vi "MCP4725_with_GraphforLoop.vi"() -> ()   [LabVIEW 2017]
uses:
  <vilib>/MakerHub/LINX/Public/Peripherals/Analog/Analog Read N Chans.vi
  <vilib>/MakerHub/LINX/Public/Peripherals/Analog/Analog Read 1 Chan.vi
  <vilib>/MakerHub/LINX/Private/Local IO/LinxI2cWrite.vi
  <vilib>/MakerHub/LINX/Public/Utilities/Check Channel.vi
  <vilib>/MakerHub/LINX/Private/Local IO/LinxAnalogRead.vi
  <vilib>/MakerHub/LINX/Public/Utilities/Open Serial.vi
  <vilib>/MakerHub/LINX/Private/Utilties/Generate Error.vi
  <vilib>/Utility/file.llb/Write Delimited Spreadsheet (DBL).vi
  <vilib>/MakerHub/LINX/LMH-LINX.lvlib
panel:
  in  "stop":bool
  out "Reader Name":string
  in  "Reading Arduino\nSerial Port":refnum<visa-resource-name>="N/A"
  in  "Save Data":bool
  out "XY Graph 2":cluster{dbl[], dbl[]}[](graph)
  out "XY Graph":cluster{dbl[], dbl[]}(graph)
  out "Voltage on Analog Channel":dbl(knob) scale=0.0..75.0
  out "Current Value written to \nDAC  input":u16
  out "Device Name":string
  out "Error Out":errorcluster
  in  "Data Collection\nTime  Interval (ms)":u32
  in  "Arduino \nSerial Port":refnum<visa-resource-name>="N/A"
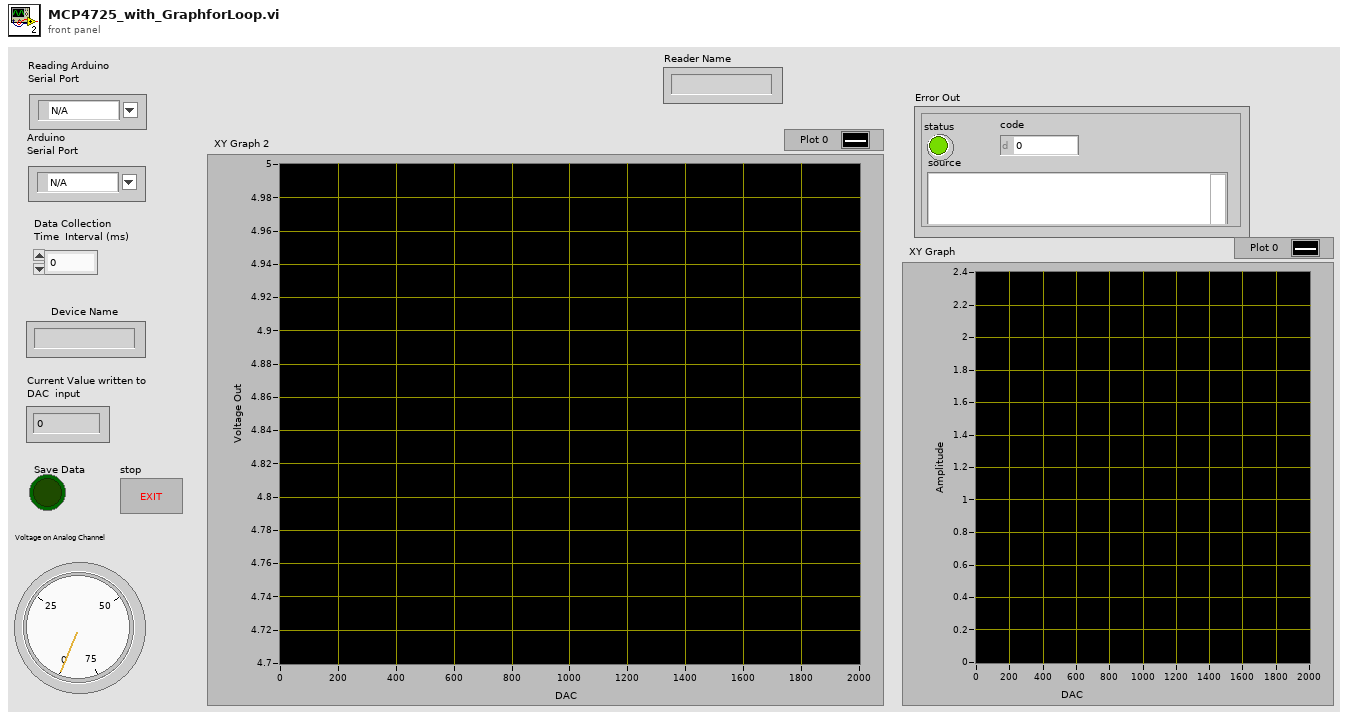
[diagram p1: front panel]
types:
  T1 = typedef "LMH-LINX.lvlib/LINX Ref.ctl" = cluster{"IO":T2, "Interface":T3, "LINX Device Config":T4}
  T2 = typedef "LMH-LINX.lvlib/Platform.ctl" = enum16{"Remote", "Local"}
  T3 = typedef "LMH-LINX.lvlib/Interface.ctl" = enum16{"Serial", "TCP"}
  T4 = typedef "LMH-LINX.lvlib/Device.lvlib/LINX Device Config.ctl" = cluster{"Interface":T3, "COM Port":refnum<visa-resource-name>, "TCP Configuration":T5, "Device Family":u8, "Device ID":u8, "Device Name":string, "TCP Ref":refnum<k5>, "Channels":T6}
  T5 = typedef "LMH-LINX.lvlib/Device.lvlib/TCP Config.ctl" = cluster{"IP Address":string, "Port":u16}
  T6 = typedef "LMH-LINX.lvlib/Channels.ctl" = cluster{"DI":u8[], "DO":u8[], "AI":u8[], "AO":u8[], "PWM":u8[], "QE":u8[], "UART":u8[], "I2C 2":u8[], "SPI":u8[], "CAN":u8[], "Servo":u8[], "AI Ref (V)":dbl, "AI Resolution (Bits)":u8, "AO Ref (V)":dbl, "AO Resolution (Bits)":u8}
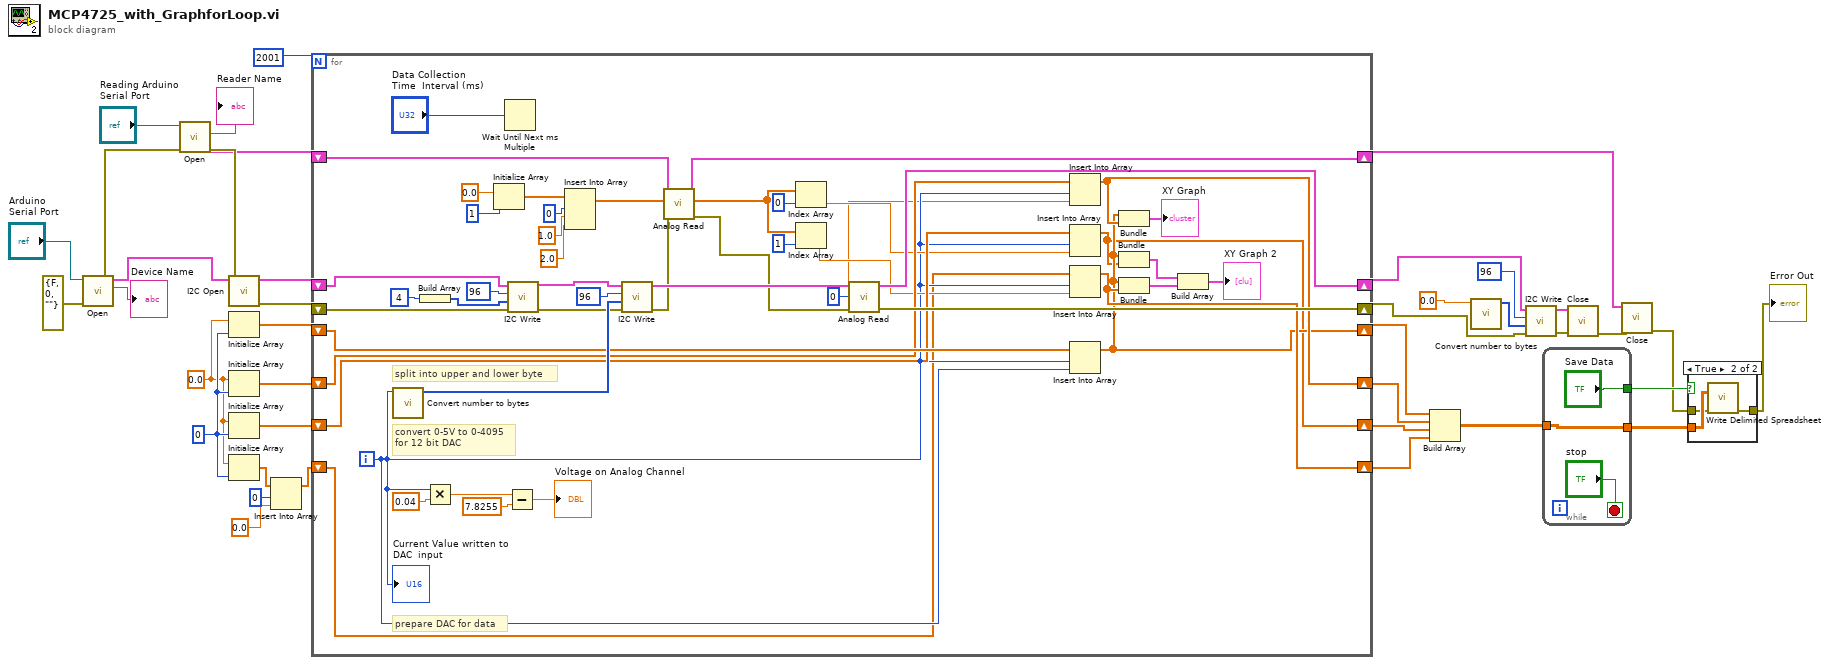
[diagram p0: block diagram]
diagram:
  w24 = 0.0 ("element")
  w25 = 0 ("dimension size")
  n1 = call-poly <vilib>:"Open.vi"("Error In"=errorcluster {"status"=FALSE, "code"=0, "source"=""}, "Serial Port"="Arduino \nSerial Port") -> ("Error Out"=w9:errorcluster, "Device Name"=→"Device Name":string, "LINX Resource"=w38:T1)  [unwired: 7 in]
  n2 = call-poly <vilib>:"Open.vi"("Error In"=w9, "Serial Port"="Reading Arduino\nSerial Port") -> ("Error Out"=w8:errorcluster, "Device Name"=→"Reader Name":string, "LINX Resource"=w6:T1)  [unwired: 7 in]
  n3 = call <vilib>:"I2C Open.vi"("Error In"=w8, "LINX Resource"=w38) -> ("Error Out"=w35:errorcluster, "LINX Resource"=w36:T1)  [unwired: 8 in]
  n4 = Initialize Array(w24, w25) -> (w33:dbl[])
  n5 = Initialize Array(w24, w25) -> (w32:dbl[])
  n6 = Initialize Array(w24, w25) -> (w23:dbl[])
  n7 = Initialize Array(w24, w25) -> (w14:dbl[])
  n8 = Insert Into Array(array=w14, index=0, new element=0.0 ("new element/subarray")) -> (w11:dbl[])
  n9 = for {
    N: 2001 -> [_]
    shift-right: [w78] -> w18
    shift-left: w36 -> [w87]
    shift-right: [w77] -> w16
    shift-left: w35 -> [w86]
    shift-right: [w57] -> w22
    shift-left: w33 -> [w75]
    shift-right: [w62] -> w21
    shift-left: w32 -> [w74]
    shift-right: [w56] -> w20
    shift-left: w23 -> [w61]
    shift-right: [w58] -> w19
    shift-left: w11 -> [w49]
    shift-right: [w46] -> w3
    shift-left: w6 -> [w47]
    i -> [w52]
    # "prepare DAC for data"
    # "convert 0-5V to 0-4095\nfor 12 bit DAC"
    # "split into upper and lower byte"
    n10 = call "Convert number to bytes.vi"("Numeric"=w52) -> ("Array"=w84:u8[])  [unwired: 10 in]
    n11 = Build Array(u8 4) -> (w80:u8[])
    n12 = Multiply(x=w52, y=0.04) -> (x*y=w65:dbl)
    n13 = Initialize Array(0.0 ("element"), 1 ("dimension size")) -> (w68:dbl[])
    n14 = Wait Until Next ms Multiple(millisecond multiple="Data Collection\nTime  Interval (ms)") -> ()  [unwired: 1 out]
    n15 = Subtract(x=w65, y=7.8255) -> (x-y=→"Voltage on Analog Channel":dbl)
    n16 = call <vilib>:"I2C Write.vi"("Error In"=w86, "Data"=w80, "I2C Slave Address (0)"=u8 96, "LINX Resource"=w87) -> ("Error Out"=w72:errorcluster, "LINX Resource"=w71:T1)  [unwired: 6 in]
    n17 = Insert Into Array(array=w68, index=0, new element #1=1.0 ("new element/subarray"), new element #2=2.0 ("new element/subarray")) -> (w40:dbl[])
    n18 = call <vilib>:"I2C Write.vi"("Error In"=w72, "Data"=w84, "I2C Slave Address (0)"=u8 96, "LINX Resource"=w71) -> ("Error Out"=w43:errorcluster, "LINX Resource"=w79:T1)  [unwired: 6 in]
    n19 = call-poly <vilib>:"Analog Read.vi"("Error In"=w43, "AI Channel(s)"=w40, "LINX Resource"=w47) -> ("Error Out"=w42:errorcluster, "Voltages"=w45:dbl[], "LINX Resource"=w46:T1)  [unwired: 5 in, 1 out]
    n20 = Index Array(array=w45, index=0) -> (element=w60:dbl)
    n21 = Index Array(array=w45, index=1) -> (element=w59:dbl)
    n22 = call-poly <vilib>:"Analog Read.vi"("Error In"=w42, "Analog Channel"=u8 0, "LINX Resource"=w79) -> ("Error Out"=w77:errorcluster, "Voltage"=w44:dbl, "LINX Resource"=w78:T1)  [unwired: 5 in, 1 out]
    n23 = Insert Into Array(array=w74, index=w52, new element=w44) -> (w62:dbl[])
    n24 = Insert Into Array(array=w61, index=w52, new element=w60) -> (w56:dbl[])
    n25 = Insert Into Array(array=w49, index=w52, new element=w59) -> (w58:dbl[])
    n26 = Insert Into Array(array=w75, index=w52, new element=w52) -> (w57:dbl[])
    n27 = Bundle(w57, w62) -> (→"XY Graph":cluster{dbl[], dbl[]})  [unwired: 1 in]
    n28 = Bundle(w57, w56) -> (w54:cluster{dbl[], dbl[]})  [unwired: 1 in]
    n29 = Bundle(w57, w58) -> (w55:cluster{dbl[], dbl[]})  [unwired: 1 in]
    n30 = Build Array(w54, w55) -> (→"XY Graph 2":cluster{dbl[], dbl[]}[])
    "Current Value written to \nDAC  input" <- w52
  }
  n31 = Build Array(w22, w21, w20, w19) -> (w2:dbl[][])
  n32 = call "Convert number to bytes.vi"("Numeric"=0.0) -> ("Array"=w29:u8[])  [unwired: 10 in]
  n33 = call <vilib>:"I2C Write.vi"("Error In"=w16, "Data"=w29, "I2C Slave Address (0)"=u8 96, "LINX Resource"=w18) -> ("Error Out"=w28:errorcluster, "LINX Resource"=w27:T1)  [unwired: 6 in]
  n34 = while {
    tunnel: ["Save Data"] -> w17
    tunnel: w2 -> [w88]
    tunnel: [w88] -> w1
    stop <- "stop" stop-if-true
  }
  n35 = call <vilib>:"Close.vi"("Error In"=w28, "LINX Resource"=w27) -> ("Error Out"=w5:errorcluster)  [unwired: 9 in]
  n36 = call <vilib>:"Close.vi"("Error In"=w5, "LINX Resource"=w3) -> ("Error Out"=w4:errorcluster)  [unwired: 9 in]
  n37 = case shown="True" w17 {
    tunnel: [w91 w94] -> w15
    tunnel: w4 -> [w91 w92]
    tunnel: w1 -> [_ w93]
    frame False {
    }
    frame True {
      n38 = call-poly <vilib>:"Write Delimited Spreadsheet.vi"("2D data"=w93, "error in (no error)"=w92) -> ("error out"=w94:errorcluster)  [unwired: 12 in, 1 out]
    }
  }
  "Error Out" <- w15
